vi "Set Mouse Icon.vi"(8 "error in (no error)":errorcluster, 10 "icon":u16, 11 "Xinformation In":T1) -> (0 "error out":errorcluster, 3 "Xinformation Out":T1)   [LabVIEW 2020, in "Overview XControl.xctl"]
doc: "Sets the mouse cursor to the [index] value. Set cursor to 0 to let labview handle default cursor icon"
uses:
  Overview XControl.xctl
  <vilib>/Utility/cursorutil.llb/Set Cursor (Icon Pict).vi
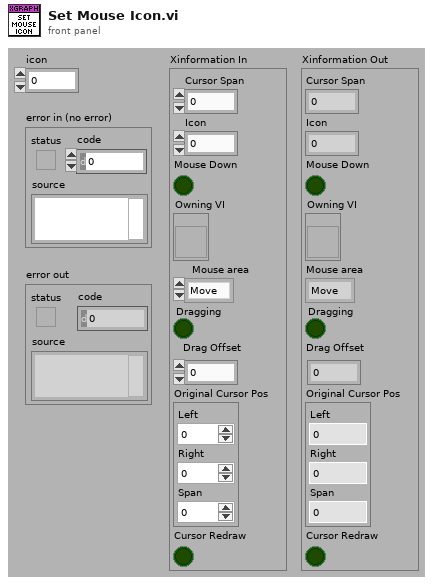
[diagram p1: front panel]
types:
  T1 = cluster{"Cursor Span":dbl, "Icon":u16, "Mouse Down":bool, "Owning VI":refnum<vi>, "Mouse area":enum16{"Move", "left cursor", "right cursor", "none"}, "Dragging":bool, "Drag Offset":dbl, "Original Cursor Pos":cluster{"Left":dbl, "Right":dbl, "Span":dbl}, "Cursor Redraw":bool}
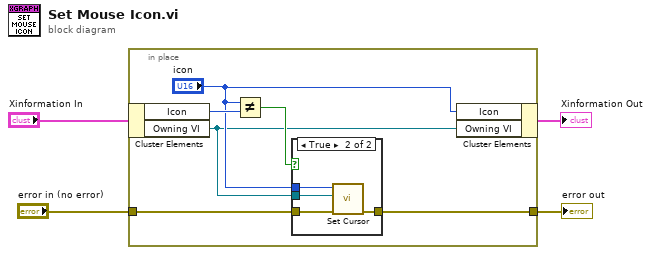
[diagram p0: block diagram]
diagram:
  n1 = in-place {
    in-place-border: "error in (no error)" -> [w6]
    in-place-border: [w5] -> w1
    n2 = in-place-cluster #1("Xinformation In") -> ("Icon"=w10:u16, "Owning VI"=w7:refnum<vi>)
    n3 = Not Equal?(x="icon", y=w10) -> (x != y?=w9:bool)
    n4 = case shown="True" w9 {
      tunnel: "icon" -> [_ w15]
      tunnel: w7 -> [_ w14]
      tunnel: w6 -> [w11 w13]
      tunnel: [w11 w12] -> w5
      frame False {
      }
      frame True {
        n5 = call-poly <vilib>:"Set Cursor.vi"("error in (no error)"=w13, "VI reference (current VI)"=w14, "icon"=w15) -> ("error out"=w12:errorcluster)  [unwired: 7 in, 1 out]
      }
    }
    n6 = in-place-cluster #1("Icon"="icon", "Owning VI"=w7) -> (→"Xinformation Out":T1)
  }
  "error out" <- w1
